vi "Open Right Splitter Pos.vi"(8 "error in (no error)":errorcluster, 11 "This VI":refnum<vi>) -> (0 "error out":errorcluster)   [LabVIEW 2014]
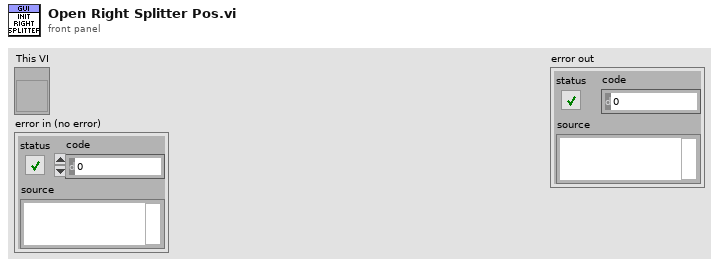
[diagram p1: front panel]
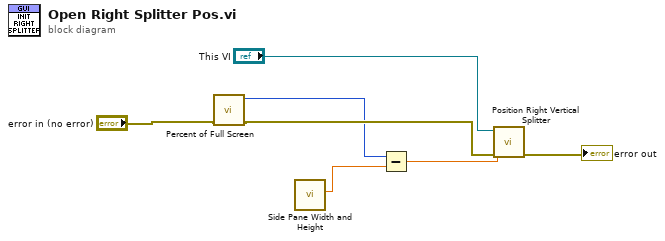
[diagram p0: block diagram]
diagram:
  n1 = call "Percent of Full Screen.vi"("error in (no error)"="error in (no error)") -> ("error out"=w4:errorcluster, "Right"=w3:i16)  [unwired: 8 in, 1 out]
  n2 = call "Side Pane Width and Height.vi"() -> ("Width"=w1:dbl)  [unwired: 9 in, 2 out]
  n3 = Subtract(x=w3, y=w1) -> (x-y=w2:dbl)
  n4 = call "Position Right Vertical Splitter.vi"("error in (no error)"=w4, "Splitter Position"=w2, "This VI"="This VI") -> ("error out"=→"error out":errorcluster)  [unwired: 8 in]
